vi "Position B.vi"(8 "error in (no error)":errorcluster, 11 "VICI Electronic Actuator":T1) -> (0 "error out":errorcluster, 1 "Initialized":bool, 3 "VICI Electronic Actuator":T1)   [LabVIEW 2018, in "VICI Electronic Actuator.lvlib"]
uses:
  D-O Module Folder/DIO Valve/VICI Electronic Actuator.lvlib
  VICI Electronic Actuator Settings.ctl
  <vilib>/Instr/_visa.llb/VISA Configure Serial Port (Instr).vi
panel:
  out "No Pump Connected 2":bool
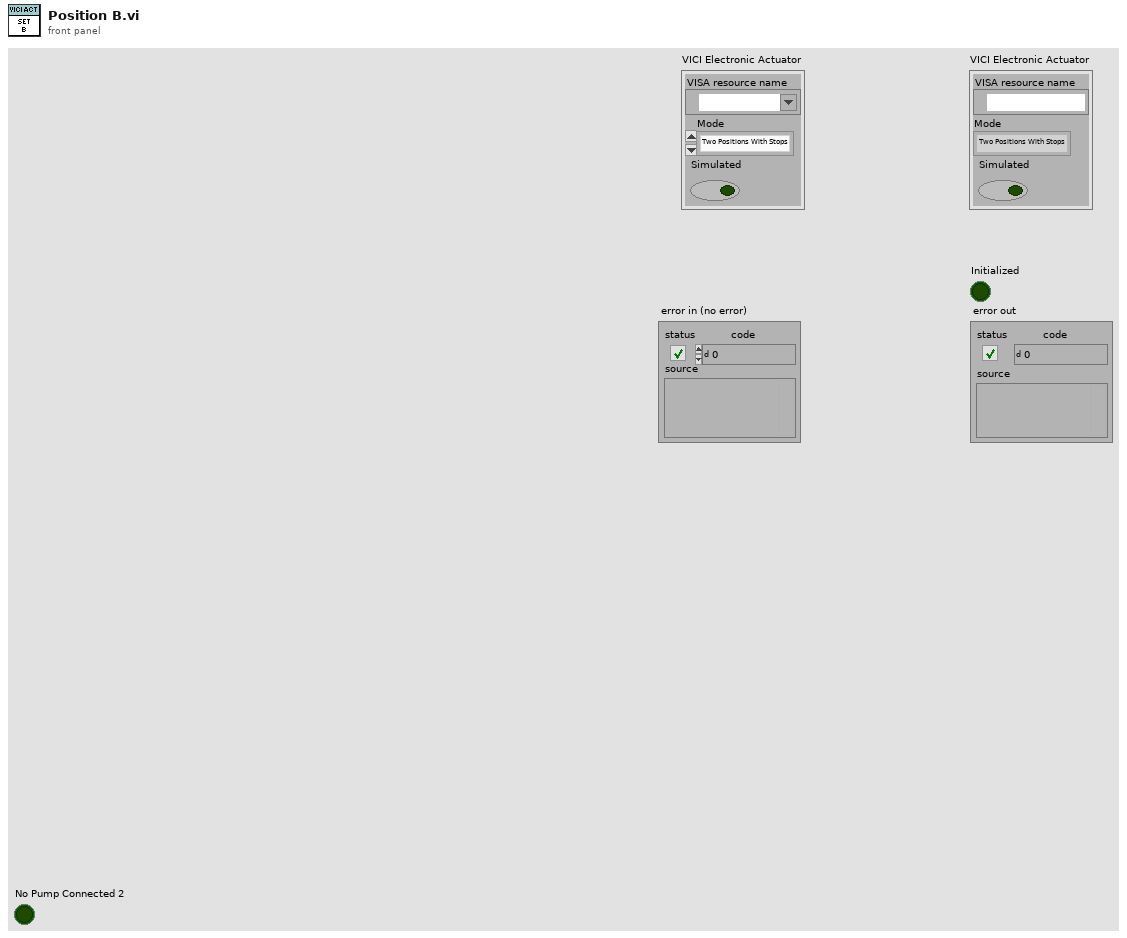
[diagram p1: front panel]
types:
  T1 = typedef "VICI Electronic Actuator.lvlib/VICI Electronic Actuator Settings.ctl" = cluster{"VISA resource name":refnum<visa-resource-name>, "Mode":enum16{"Two Positions With Stops", "Two Positions Without Stops", "Mutiposition"}, "Simulated":bool}
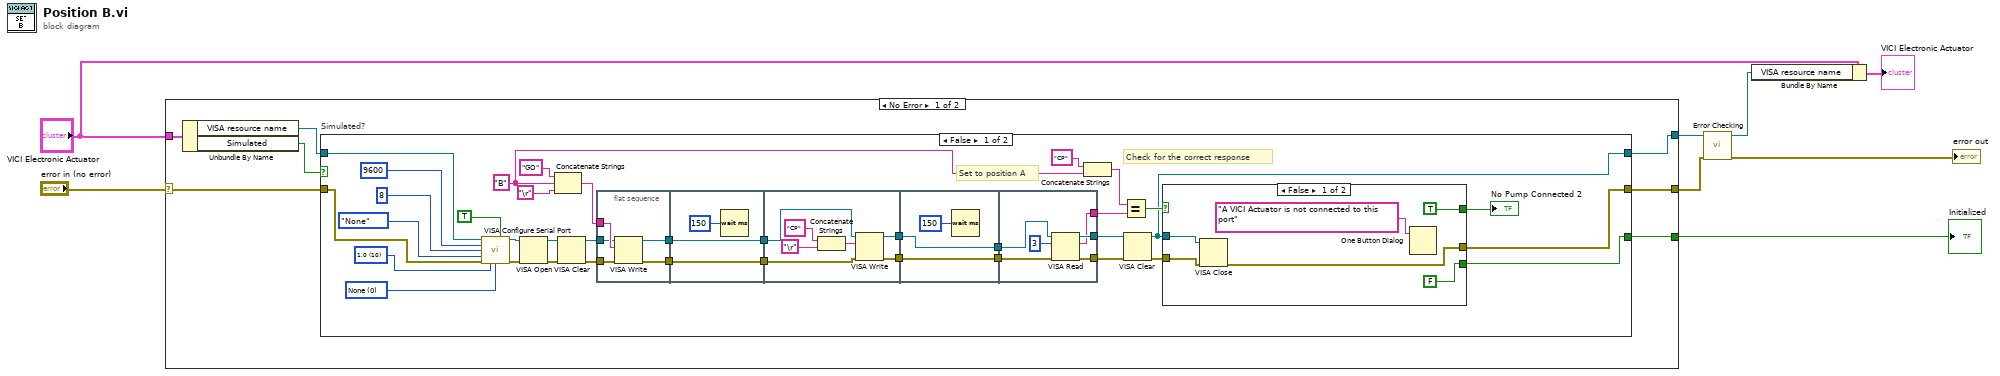
[diagram p0: block diagram]
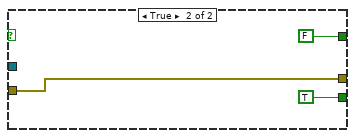
[diagram p2: hidden frame]
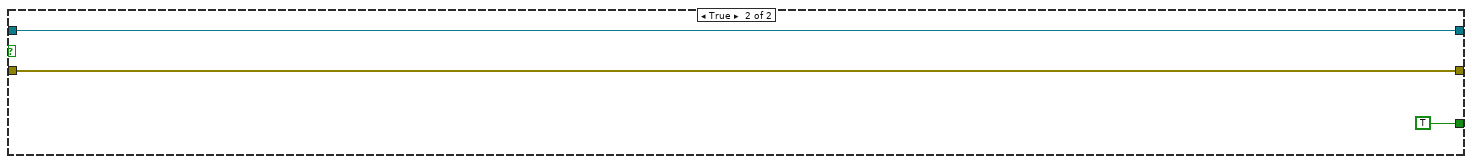
[diagram p3: hidden frame]
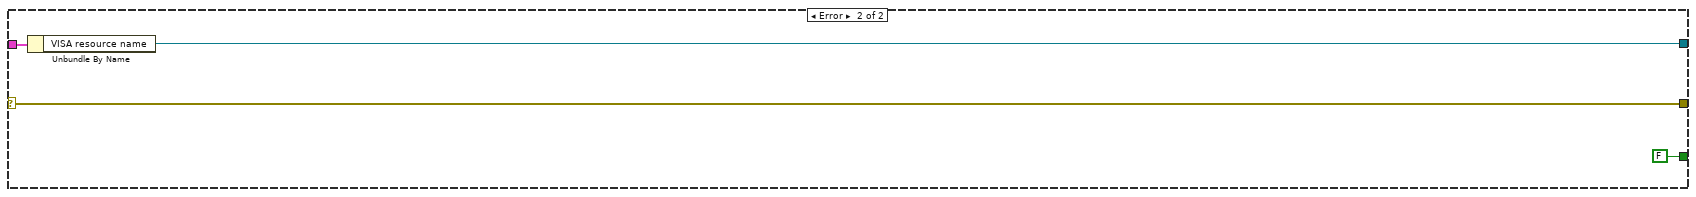
[diagram p4: hidden frame]
diagram:
  n1 = case shown="No Error" "error in (no error)" {
    selector: "error in (no error)" -> [w15 w92]
    tunnel: "VICI Electronic Actuator" -> [w12 w91]
    tunnel: [w13 w92] -> w7
    tunnel: [w10 w90] -> w8
    tunnel: [w9 FALSE] -> w2
    frame No Error {
      n2 = Unbundle By Name(w12) -> ("VISA resource name"=w11:refnum<visa-resource-name>, "Simulated"=w14:bool)
      n3 = case "Simulated?" shown="False" w14 {
        tunnel: w15 -> [w46 w88]
        tunnel: [w36 w88] -> w13
        tunnel: [w42 w87] -> w10
        tunnel: w11 -> [w44 w87]
        tunnel: [w35 TRUE] -> w9
        frame False {
          w22 = "B"
          w48 = u16 0 items=["None", "XON/XOFF", "RTS/CTS", "XON/XOFF & RTS/CTS", "DTR/DSR", "XON/XOFF & DTR/DSR"] ("flow control (0:none)")
          w49 = u16 10 items=["1.0"=10, "1.5"=15, "2.0"=20] ("stop bits (10: 1 bit)")
          # "Check for the correct response"
          # "Set to position A"
          n4 = call-poly "VISA Configure Serial Port"("VISA resource name"=w44, "Enable Termination\nChar (T)"=TRUE ("Enable Termination\nChar (T)"), "baud rate (9600)"=u32 9600, "data bits (8)"=u16 8, "parity (0:none)"=enum16{"None", "Odd", "Even", "Mark", "Space"}."None", "error in (no error)"=w46, "stop bits (10: 1 bit)"=w49, "flow control (0:none)"=w48) -> ("VISA resource name out"=w45:refnum<visa-resource-name>, "error out"=w47:errorcluster)  [unwired: 6 in]
          n5 = VISA Open(error in (no error)=w47, VISA resource name=w45) -> (VISA resource name=w41:refnum<visa-resource-name>, error out=w40:errorcluster)  [unwired: 3 in]
          n6 = Concatenate Strings("GO" ("string"), w22, "\r") -> (w26:string)
          n7 = VISA Clear(VISA resource name=w41, error in (no error)=w40) -> (VISA resource name out=w25:refnum<visa-resource-name>, error out=w27:errorcluster)
          n8 = flat-sequence {
            tunnel: [w53] -> w34
            tunnel: [w54] -> w33
            tunnel: w27 -> [w57]
            tunnel: w26 -> [w56]
            tunnel: w25 -> [w55]
            tunnel: [w59] -> w21
            tunnel: w34 -> [w59]
            tunnel: w33 -> [w58]
            tunnel: [w58] -> w20
            tunnel: w21 -> [w67]
            tunnel: [w65] -> w19
            tunnel: w20 -> [w66]
            tunnel: [w64] -> w17
            tunnel: w19 -> [w70]
            tunnel: [w70] -> w18
            tunnel: w17 -> [w69]
            tunnel: [w69] -> w16
            tunnel: [w76] -> w28
            tunnel: [w75] -> w29
            tunnel: w18 -> [w73]
            tunnel: w16 -> [w72]
            tunnel: [w71] -> w31
            frame #0 {
              n9 = VISA Write(VISA resource name=w55, write buffer=w56, error in (no error)=w57) -> (VISA resource name out=w53:refnum<visa-resource-name>, error out=w54:errorcluster)  [unwired: 1 out]
            }
            frame #1 {
              n10 = Wait (ms)(milliseconds to wait=u32 150) -> ()  [unwired: 1 out]
            }
            frame #2 {
              n11 = Concatenate Strings("CP" ("write buffer"), "\r") -> (w62:string)
              n12 = VISA Write(VISA resource name=w67, write buffer=w62, error in (no error)=w66) -> (VISA resource name out=w65:refnum<visa-resource-name>, error out=w64:errorcluster)  [unwired: 1 out]
            }
            frame #3 {
              n13 = Wait (ms)(milliseconds to wait=u32 150) -> ()  [unwired: 1 out]
            }
            frame #4 {
              n14 = VISA Read(VISA resource name=w73, byte count=u32 3, error in (no error)=w72) -> (VISA resource name out=w75:refnum<visa-resource-name>, read buffer=w71:string, error out=w76:errorcluster)  [unwired: 1 out]
            }
          }
          n15 = Concatenate Strings("CP" ("string"), w22) -> (w30:string)
          n16 = Equal?(x=w30, y=w31) -> (x = y?=w43:bool)
          n17 = VISA Clear(VISA resource name=w29, error in (no error)=w28) -> (VISA resource name out=w42:refnum<visa-resource-name>, error out=w37:errorcluster)
          n18 = case shown="False" w43 {
            tunnel: w42 -> [w81 _]
            tunnel: w37 -> [w80 w84]
            tunnel: [TRUE FALSE] -> w38
            tunnel: [w78 w84] -> w36
            tunnel: [FALSE TRUE] -> w35
            frame False {
              n19 = VISA Close(VISA resource name=w81, error in (no error)=w80) -> (error out=w78:errorcluster)
              n20 = One Button Dialog(message="A VICI Actuator is not connected to this port") -> ()  [unwired: 1 in, 1 out]
            }
            frame True {
            }
          }
          "No Pump Connected 2" <- w38
        }
        frame True {
        }
      }
    }
    frame Error {
      n21 = Unbundle By Name(w91) -> ("VISA resource name"=w90:refnum<visa-resource-name>)
    }
  }
  "Initialized" <- w2
  n22 = call "Error Checking.vi"("error in (no error)"=w7, "VISA resource name"=w8) -> ("error out"=→"error out":errorcluster, "VISA resource name"=w6:refnum<visa-resource-name>)  [unwired: 7 in, 1 out]
  n23 = Bundle By Name(cluster="VICI Electronic Actuator", "VISA resource name"=w6) -> (→"VICI Electronic Actuator":T1)
